vi "Edit Config.vi"(8 "error in (no error)":errorcluster, 11 "Multiple Queries in":refnum<class "Multiple Queries.lvclass">) -> (0 "error out":errorcluster, 3 "Multiple Queries out":refnum<class "Multiple Queries.lvclass">)   [LabVIEW 2015, in "Multiple Queries.lvclass"]
doc: "Single Query.lvclass:Edit Config.vi\n\nThis VI is used to edit the Single Query configuration parameters.\n\nInstrument Communication Module Version 1.0\nDecember, 2017 Original Code Consulting David Thomson\n www.originalcode.com"
uses:
  Multiple Queries.lvclass
  Multiple Queries Config.ctl
  Controls/ICM Class Editor State.ctl
  Controls/ICM Editor Command.ctl
  Multiple Queries.lvclass/Multiple Queries.ctl
panel:
  in  "Save":bool
  in  "Revert":bool
  in  "Multiple Queries Config":T1
  # "The Multiple Queries class is used more than one Query/Response\nis required to obtain all the desired data channels from an Instrument."
  # "These parameters are displayed using the \"\\\" codes display.\nUse \\s for space, \\r for <CR>, \\n for <LF>, etc."
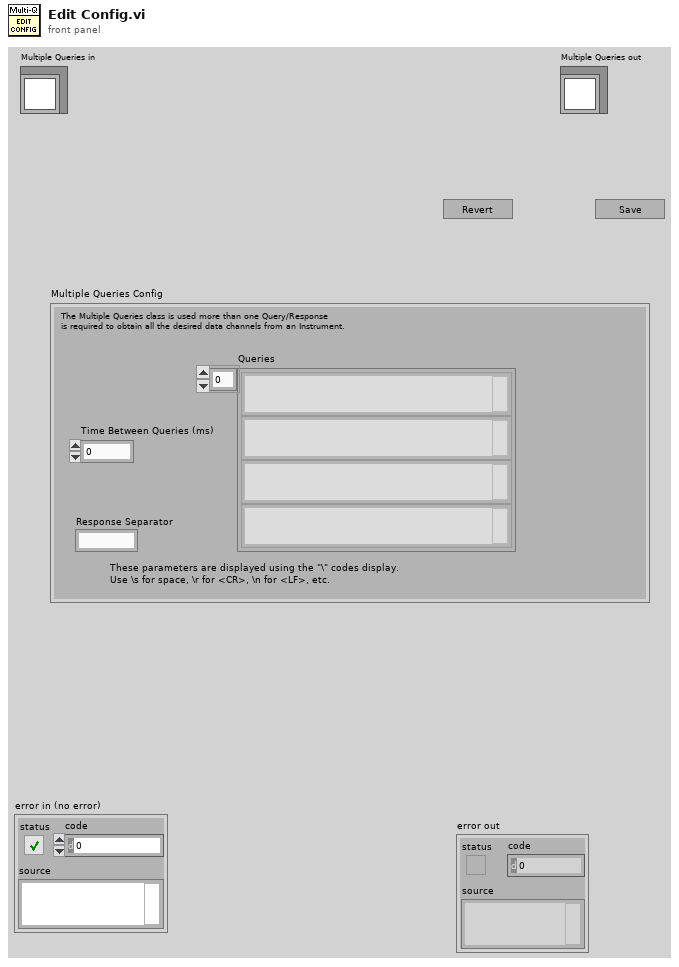
[diagram p1: front panel]
types:
  T1 = typedef "Multiple Queries.lvclass/Multiple Queries Config.ctl" = cluster{"Response Separator":string, "Queries":string[], "Time Between Queries (ms)":u32}
  T2 = typedef "ICM Editor Command.ctl" = enum16{"No-op", "Exit"}
  T3 = typedef "ICM Class Editor State.ctl" = enum16{"Init", "Wait", "Write", "Read", "Display", "Set Flashing", "Error", "Stop"}
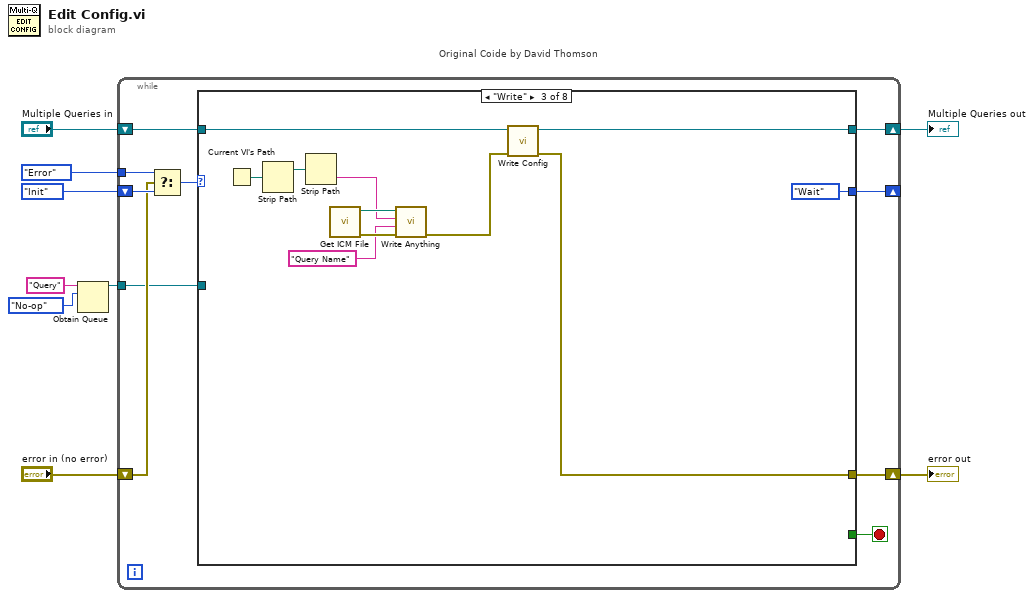
[diagram p0: block diagram]
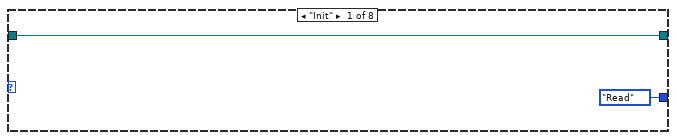
[diagram p2: hidden frame]
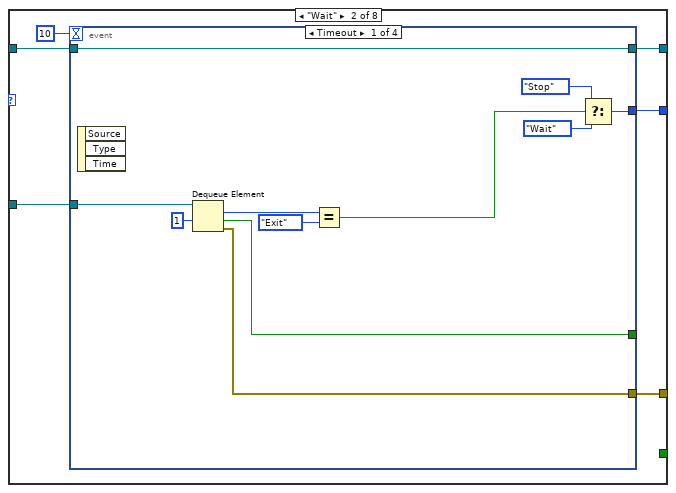
[diagram p3: hidden frame]
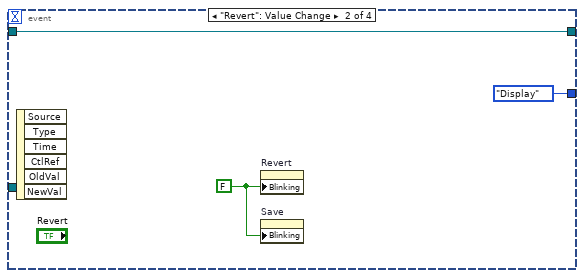
[diagram p4: hidden frame]
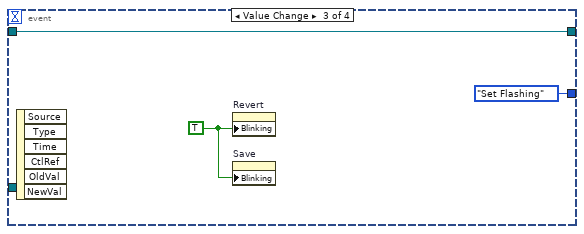
[diagram p5: hidden frame]
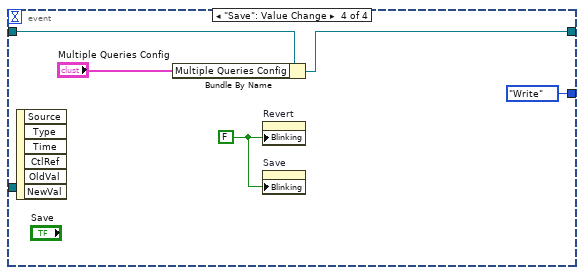
[diagram p6: hidden frame]
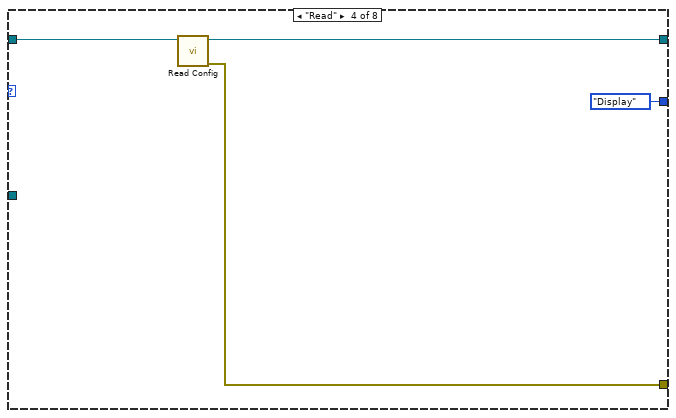
[diagram p7: hidden frame]
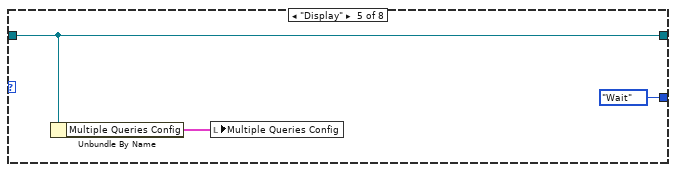
[diagram p8: hidden frame]
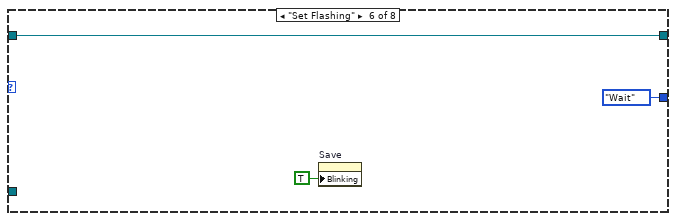
[diagram p9: hidden frame]
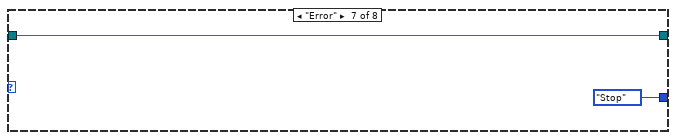
[diagram p10: hidden frame]
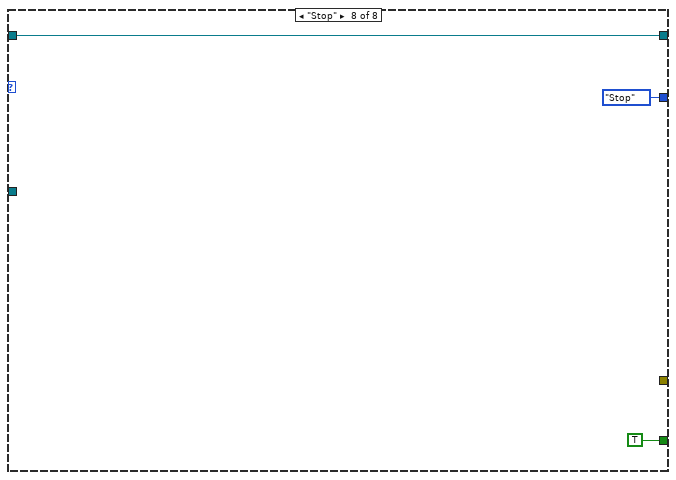
[diagram p11: hidden frame]
diagram:
  n1 = Obtain Queue(name (unnamed)="Query", element data type=ICM_Editor_Command."No-op" ("Editor Command")) -> (queue out=w1:refnum<queue>)  [unwired: 3 in, 2 out]
  n2 = while "Original Coide by David Thomson" {
    shift-right: [w19] -> w8
    shift-left: "Multiple Queries in" -> [w18]
    shift-right: [w12] -> _
    shift-left: ICM_Class_Editor_State."Init" ("Config State") -> [w16]
    shift-right: [w11] -> w6
    shift-left: "error in (no error)" -> [w14]
    tunnel: ICM_Class_Editor_State."Error" ("Config State") -> [w13]
    tunnel: w1 -> [w10]
    stop <- w17 stop-if-true
    n3 = Select(t=w13, s=w14, f=w16) -> (s? t:f=w15:T3)
    n4 = case shown="\"Write\"" w15 {
      tunnel: [w20 w25 w58 w63 w67 w70 w72 w75] -> w19
      tunnel: w18 -> [w20 w24 w59 w61 w67 w70 w72 w75]
      tunnel: [_ _ _ _ _ _ _ TRUE] -> w17
      tunnel: [ICM_Class_Editor_State."Read" ("Config State") w26 ICM_Class_Editor_State."Wait" ("Config State") ICM_Class_Editor_State."Display" ("Config State") ICM_Class_Editor_State."Wait" ("Config State") ICM_Class_Editor_State."Wait" ("Config State") ICM_Class_Editor_State."Stop" ("Config State") ICM_Class_Editor_State."Stop" ("Config State")] -> w12
      tunnel: [_ w22 w57 w64 _ _ _ _] -> w11
      tunnel: w10 -> [_ w23 _ _ _ _ _ _]
      frame "Init" {
      }
      frame "Wait" {
        n5 = event shown="[0] Timeout" {
          selector: _ -> [_ _ _ _]
          dyn-events: _ -> [_ _ _ _]
          timeout: 10 -> [_ _ _ _]
          tunnel: [w35 ICM_Class_Editor_State."Display" ("Config State") ICM_Class_Editor_State."Set Flashing" ("Config State") ICM_Class_Editor_State."Write" ("Config State")] -> w26
          tunnel: [w38 w40 w44 w46] -> w25
          tunnel: w24 -> [w38 w40 w44 w47]
          tunnel: w23 -> [w37 _ _ _]
          tunnel: [w29 _ _ _] -> w22
          tunnel: [w28 _ _ _] -> _
          event Timeout {
            n6 = event-data() -> ()  [unwired: 1 in, 3 out]
            n7 = Dequeue Element(queue=w37, timeout in ms (-1)=1) -> (element=w34:T2, timed out?=w28:bool, error out=w29:errorcluster)  [unwired: 1 in, 1 out]
            n8 = Equal?(x=w34, y=ICM_Editor_Command."Exit") -> (x = y?=w32:bool)
            n9 = Select(t=ICM_Class_Editor_State."Stop" ("Config State"), s=w32, f=ICM_Class_Editor_State."Wait" ("Config State")) -> (s? t:f=w35:T3)
          }
          event "Revert": Value Change {
            w39 = FALSE ("Blinking")
            n10 = event-data() -> ()  [unwired: 1 in, 6 out]
            n11 = property on="Revert" class="Bool"("Blinking"=w39) -> ()  [unwired: 2 in, 2 out]
            n12 = property on="Save" class="Bool"("Blinking"=w39) -> ()  [unwired: 2 in, 2 out]
          }
          event Value Change {
            w42 = TRUE ("Blinking")
            n13 = event-data() -> ()  [unwired: 1 in, 6 out]
            n14 = property on="Revert" class="Bool"("Blinking"=w42) -> ()  [unwired: 2 in, 2 out]
            n15 = property on="Save" class="Bool"("Blinking"=w42) -> ()  [unwired: 2 in, 2 out]
          }
          event "Save": Value Change {
            w45 = FALSE ("Blinking")
            n16 = event-data() -> ()  [unwired: 1 in, 6 out]
            n17 = Bundle By Name(cluster=w47, "Multiple Queries Config"="Multiple Queries Config") -> (w46:refnum<class "Multiple Queries.lvclass">)
            n18 = property on="Revert" class="Bool"("Blinking"=w45) -> ()  [unwired: 2 in, 2 out]
            n19 = property on="Save" class="Bool"("Blinking"=w45) -> ()  [unwired: 2 in, 2 out]
          }
        }
      }
      frame "Write" {
        n20 = Current VI's Path() -> (path=w56:path)
        n21 = Strip Path(path=w56) -> (stripped path=w55:path)  [unwired: 1 out]
        n22 = Strip Path(path=w55) -> (name=w51:string)  [unwired: 1 out]
        n23 = call "Get ICM File.vi"() -> ("error out"=w53:errorcluster, "ICM File"=w54:path)  [unwired: 10 in]
        n24 = call "Write Anything.vi"("Error In"=w53, "Section Name (Name of \"Anything\")"="Query Name" ("Section Name (Name of \"Anything\")"), "Anything"=w51, "Path (dialog)"=w54) -> ("Error Out"=w52:errorcluster)  [unwired: 7 in]
        n25 = call-dynamic "Write Config.vi"("error in (no error)"=w52, "Multiple Queries in"=w59) -> ("error out"=w57:errorcluster, "Multiple Queries out"=w58:refnum<class "Multiple Queries.lvclass">)  [unwired: 8 in]
      }
      frame "Read" {
        n26 = call-dynamic "Read Config.vi"("Multiple Queries in"=w61) -> ("error out"=w64:errorcluster, "Multiple Queries out"=w63:refnum<class "Multiple Queries.lvclass">)  [unwired: 9 in]
      }
      frame "Display" {
        n27 = Unbundle By Name(w67) -> ("Multiple Queries Config"=w66:T1)
        n28 = local write "Multiple Queries Config"(w66) -> ()
      }
      frame "Set Flashing" {
        n29 = property on="Save" class="Bool"("Blinking"=TRUE) -> ()  [unwired: 2 in, 2 out]
      }
      frame "Error" {
      }
      frame "Stop" {
      }
    }
  }
  "error out" <- w6
  "Multiple Queries out" <- w8
